vi "Spindexer_Begin.vi"   [LabVIEW 2019]
uses:
  Spindexer_Cluster.ctl
  Spindexer_mode.ctl
  Globals/Spindexer_Globals.vi
types:
  T1 = typedef "Spindexer_Cluster.ctl" = cluster{"Throttle":dbl, "Fire?":bool, "Intake recently moved?":bool, "Mode":T2, "Sensor in position? ":bool}
  T2 = typedef "Spindexer_mode.ctl" = enum16{"No-Op", "Sensing", "Intaking", "Firing(Speed Control)", "Manual"}
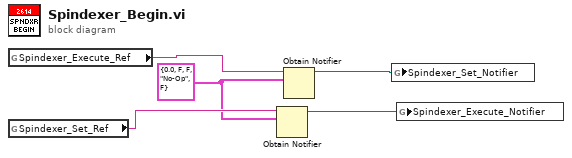
[diagram p0: block diagram]
diagram:
  w1 = T1 {"Throttle"=0.0, "Fire?"=FALSE, "Intake recently moved?"=FALSE, "Mode"=enum."No-Op", "Sensor in position? "=FALSE}
  n1 = global read "Spindexer_Globals.vi" "Spindexer_Execute_Ref"() -> (w2:string)
  n2 = global read "Spindexer_Globals.vi" "Spindexer_Set_Ref"() -> (w3:string)
  n3 = Obtain Notifier(name (unnamed)=w3, notification data type=w1) -> (notifier out=w5:refnum<notifier>)  [unwired: 2 in, 2 out]
  n4 = Obtain Notifier(name (unnamed)=w2, notification data type=w1) -> (notifier out=w4:refnum<notifier>)  [unwired: 2 in, 2 out]
  n5 = global write "Spindexer_Globals.vi" "Spindexer_Set_Notifier"(w4) -> ()
  n6 = global write "Spindexer_Globals.vi" "Spindexer_Execute_Notifier"(w5) -> ()
